vi "CANOpen_Get SDOs Settings.vi"(8 "error in":errorcluster, 11 "Device Ref in":T2 format="%.0x") -> (0 "error out":errorcluster, 2 "SDOs":T1[](array[typedef]) {"Block Data" format="%.0x"}, 3 "Device Ref out":T2 format="%.0x")   [LabVIEW 2021, in "CANOpen Addon Engine.lvlib"]
uses:
  CANOpen Addon Engine.lvlib
  <vilib>/NI VeriStand/Custom Device API/Custom Device Item Ref.ctl
  Shared/CANOpen_SDO Settings.ctl
  Shared/CANOpen Addon GUID Lookup Global.vi
  <vilib>/NI VeriStand/Custom Device Tools/Custom Device Utility Library/NI VeriStand - Search for Item by GUID.vi
  <vilib>/NI VeriStand/Custom Device API/Get Item Property (Variant).vi
  <vilib>/NI VeriStand/Custom Device Tools/Custom Device Utility Library/Custom Device Utility Library.lvlib
  Shared/CANOpen Addon Shared.lvlib
  <vilib>/NI VeriStand/Custom Device API/Custom Device API.lvlib
panel:
  # "LSB"
  # "MSB"
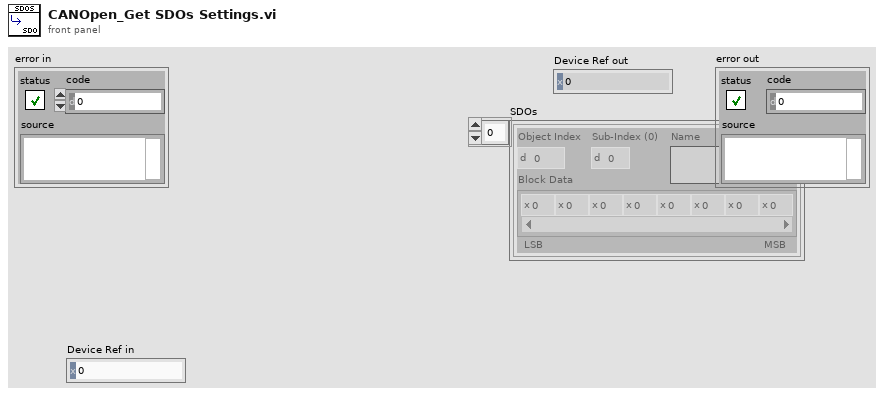
[diagram p1: front panel]
types:
  T1 = typedef "CANOpen Addon Shared.lvlib/CANOpen_SDO Settings.ctl" = cluster{"Object Index":u16, "Sub-Index (0)":u8, "Block Data":u8[], "Name":string}
  T2 = typedef "Custom Device API.lvlib/Custom Device Item Ref.ctl" = u64
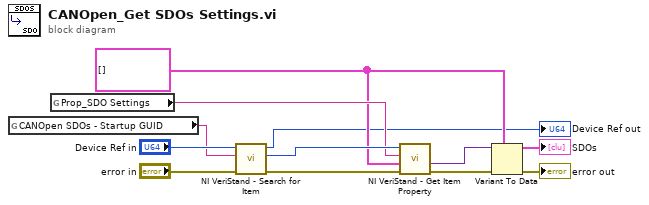
[diagram p0: block diagram]
diagram:
  w4 = T1[] [] ("SDO Parameters")
  n1 = global read "CANOpen Addon GUID Lookup Global.vi" "CANOpen SDOs - Startup GUID"() -> (w11:string)
  n2 = global read "CANOpen Addon GUID Lookup Global.vi" "Prop_SDO Settings"() -> (w7:string)
  n3 = call-poly <vilib>:"NI VeriStand - Search for Item.vi"("error in"="error in", "Item GUID"=w11, "Section Ref in"="Device Ref in") -> ("error out"=w9:errorcluster, "Item Ref"=w8:T2, "Section Ref out"=→"Device Ref out":T2)  [unwired: 5 in, 1 out]
  n4 = call-poly <vilib>:"NI VeriStand - Get Item Property.vi"("error in (no error)"=w9, "Default Value"=w4, "Property Name"=w7, "Item Ref in"=w8) -> ("error out"=w6:errorcluster, "Value"=w5:variant)  [unwired: 4 in, 2 out]
  n5 = Variant To Data(error in=w6, type=w4, Variant=w5) -> (data=→"SDOs":T1[], error out=→"error out":errorcluster)
